vi "Read Status.vi"(11 "Method Result In":refnum<class "Method Result.lvclass">) -> (1 "Glyph Index":i32=5, 2 "Status":T1, 3 "Method Result Out":refnum<class "Method Result.lvclass">)   [LabVIEW 2020, in "Method Result.lvclass"]
uses:
  Method Result.lvclass
  Assertion Result/Public/TypeDefs/Status.ctl
  Method Result.lvclass/Method Result.ctl
  Assertion Result/Assertion Result.lvclass
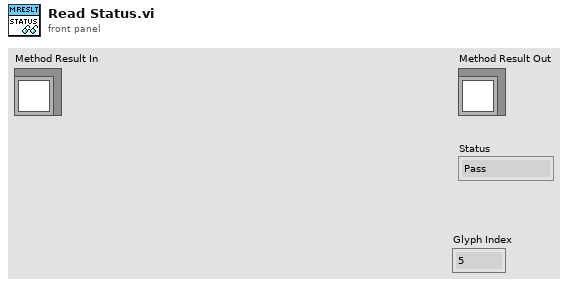
[diagram p1: front panel]
types:
  T1 = typedef "Assertion Result.lvclass/Status.ctl" = enum16{"Pass", "Fail", "Error", "Skipped", "Setup Error", "Broken", "Teardown Error"}
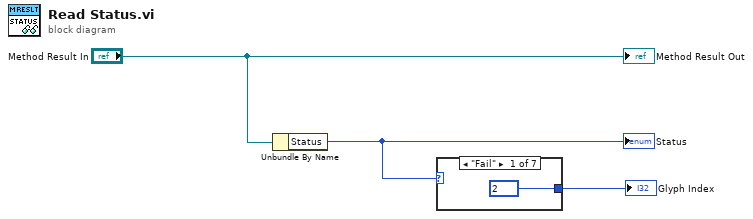
[diagram p0: block diagram]
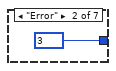
[diagram p2: hidden frame]
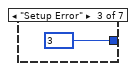
[diagram p3: hidden frame]
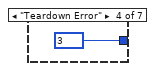
[diagram p4: hidden frame]
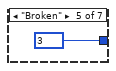
[diagram p5: hidden frame]
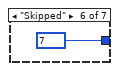
[diagram p6: hidden frame]
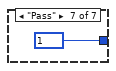
[diagram p7: hidden frame]
diagram:
  n1 = Unbundle By Name("Method Result In") -> ("Status"=w2:T1)
  "Status" <- w2
  n2 = case shown="\"Fail\"" w2 {
    tunnel: [2 ("Listbox Symbol Ring Constant") 3 ("Listbox Symbol Ring Constant") 3 ("Listbox Symbol Ring Constant") 3 ("Listbox Symbol Ring Constant") 3 ("Listbox Symbol Ring Constant") 7 ("Listbox Symbol Ring Constant") 1 ("Listbox Symbol Ring Constant")] -> w1
    frame "Fail" {
    }
    frame "Error" {
    }
    frame "Setup Error" {
    }
    frame "Teardown Error" {
    }
    frame "Broken" {
    }
    frame "Skipped" {
    }
    frame "Pass" {
    }
  }
  "Glyph Index" <- w1
  "Method Result Out" <- "Method Result In"
